vi "Set Open_(True).vi"(8 "error in (no error)":errorcluster, 10 "Open?(True)":bool, 11 "Console Reply in":refnum<class "Console Reply.lvclass">) -> (0 "error out":errorcluster, 3 "Console Reply out":refnum<class "Console Reply.lvclass">)   [LabVIEW 2015, in "EditPanel API.lvlib" / "Console Reply.lvclass"]
uses:
  Console Reply.lvclass
  Console Reply.lvclass/Console Reply.ctl
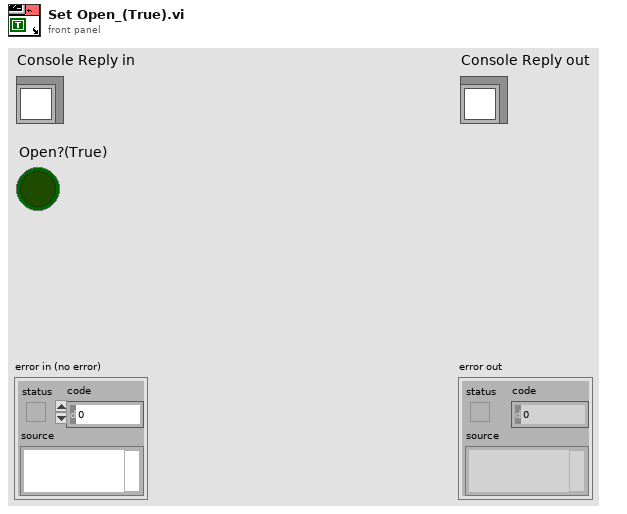
[diagram p1: front panel]
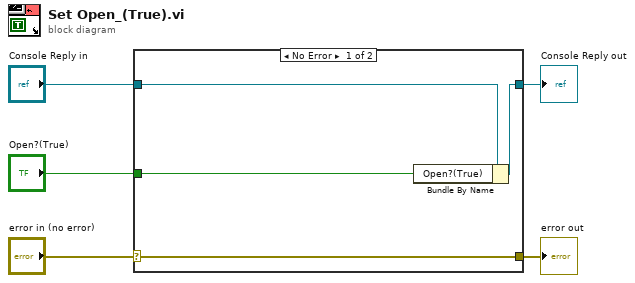
[diagram p0: block diagram]
diagram:
  n1 = case shown="No Error" "error in (no error)" {
    selector: "error in (no error)" -> [w9 w10]
    tunnel: [w9 w10] -> w4
    tunnel: [w7 w11] -> w2
    tunnel: "Console Reply in" -> [w8 w11]
    tunnel: "Open?(True)" -> [w6 _]
    frame No Error {
      n2 = Bundle By Name(cluster=w8, "Open?(True)"=w6) -> (w7:refnum<class "Console Reply.lvclass">)
    }
    frame Error {
    }
  }
  "error out" <- w4
  "Console Reply out" <- w2
